vi "配置写入.vi"(8 "error in (no error)":errorcluster caption="错误输入（无错误）") -> (0 "错误输出":errorcluster)   [LabVIEW 2016, in "斯坦道总磷总氮.lvlib"]
uses:
  <vilib>/Utility/config.llb/NI_LVConfig.lvlib
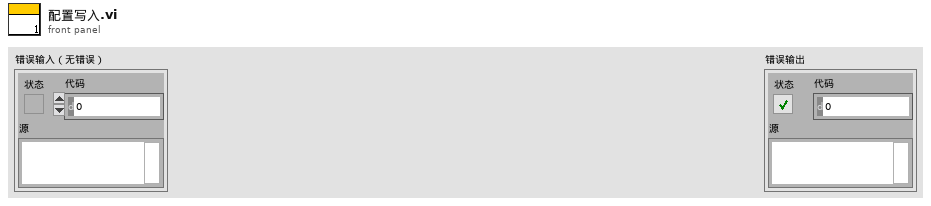
[diagram p1: front panel]
types:
  T1 = typedef "NI_LVConfig.lvlib/Config Data RefNum.ctl" = refnum<k1>
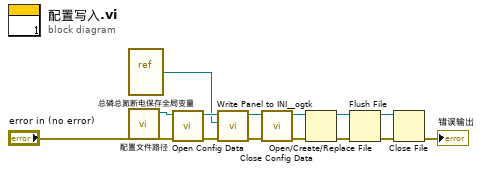
[diagram p0: block diagram]
diagram:
  n1 = vi-ref "总磷总氮断电保存全局变量.vi"() -> (w13:refnum<vi>)
  n2 = call "配置文件路径.vi"() -> ("appended path"=w1:path)  [unwired: 11 in]
  n3 = call <vilib>:"Open Config Data.vi"("error in (no error)"="error in (no error)", "configuration file path"=w1) -> ("error out"=w11:errorcluster, "refnum"=w14:T1)  [unwired: 7 in, 1 out]
  n4 = call <userlib>:"Write Panel to INI__ogtk.vi"("error in (no error)"=w11, "VI ref"=w13, "refnum"=w14) -> ("error out"=w10:errorcluster, "refnum out"=w12:T1)  [unwired: 7 in]
  n5 = call <vilib>:"Close Config Data.vi"("error in (no error)"=w10, "refnum"=w12) -> ("error out"=w5:errorcluster, "file path"=w4:path)  [unwired: 8 in]
  n6 = Open/Create/Replace File(file path (use dialog)=w4, error in=w5) -> (refnum out=w8:refnum<file>, error out=w9:errorcluster)  [unwired: 4 in, 1 out]
  n7 = Flush File(refnum=w8, error in=w9) -> (refnum out=w7:refnum<file>, error out=w6:errorcluster)
  n8 = Close File(refnum=w7, error in=w6) -> (error out=→"错误输出":errorcluster)  [unwired: 1 out]
